vi "Write value history.vi"(8 "error in (no error)":errorcluster, 10 "value history":cluster{"time as number":dbl, "Value":dbl}[](array[cluster]), 11 "PrepLineObject in":refnum<class "PrepLineObject.lvclass">) -> (0 "error out":errorcluster, 3 "PrepLineObject out":refnum<class "PrepLineObject.lvclass">)   [LabVIEW 2018, in "PrepLineObject.lvclass"]
uses:
  PrepLineObject.lvclass
  PrepLineObject.lvclass/PrepLineObject.ctl
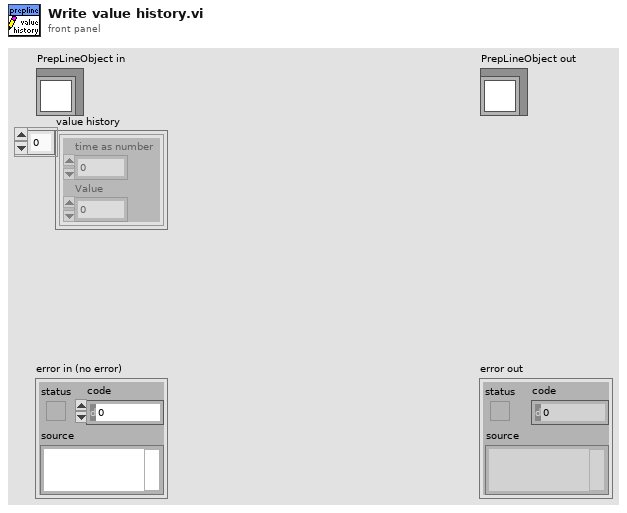
[diagram p1: front panel]
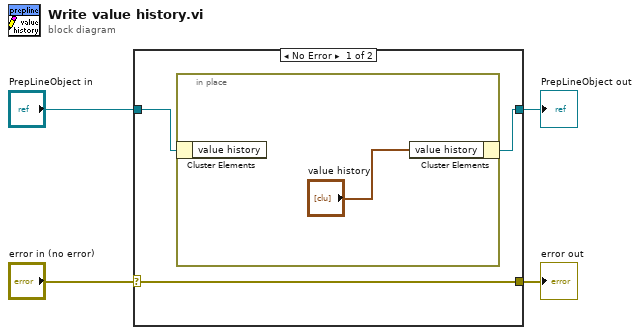
[diagram p0: block diagram]
diagram:
  n1 = case shown="No Error" "error in (no error)" {
    selector: "error in (no error)" -> [w7 w9]
    tunnel: [w7 w9] -> w3
    tunnel: [w5 w10] -> w1
    tunnel: "PrepLineObject in" -> [w6 w10]
    frame No Error {
      n2 = in-place {
        n3 = in-place-cluster #1(w6) -> ()  [unwired: 1 out]
        n4 = in-place-cluster #1("value history"="value history") -> (w5:refnum<class "PrepLineObject.lvclass">)
      }
    }
    frame Error {
    }
  }
  "error out" <- w3
  "PrepLineObject out" <- w1
